vi "PositionControlwithGCompensation.vi"() -> ()   [LabVIEW 2019]
uses:
  <vilib>/myRIO/Common/Instrument Driver Framework/myRIO v1.0/Encoder/typedefs/Encoder Signal Mode.ctl
  <vilib>/myRIO/Instrument Drivers/Onboard IO/Encoder/typedefs/Encoder Reference.ctl
  <vilib>/myRIO/Common/Instrument Driver Framework/Utilities/typedefs/myRIO Generic Hardware Reference.ctl
  <vilib>/myRIO/Common/Instrument Driver Framework/Utilities/typedefs/Hardware Version Enum.ctl
  <vilib>/myRIO/Common/Instrument Driver Framework/Utilities/typedefs/myRIO v1.0 Reference.ctl
  <vilib>/myRIO/Common/Instrument Driver Framework/Utilities/typedefs/Generic FPGA Reference.ctl
  <vilib>/myRIO/Common/Instrument Driver Framework/myRIO v1.0/Encoder/typedefs/Encoder Channels Enum.ctl
  <vilib>/myRIO/Common/Instrument Driver Framework/myRIO v1.0/Encoder/typedefs/Encoder Configuration v1.0.ctl
  <vilib>/userDefined/High Color/nirio_resource_hc.ctl
  <vilib>/myRIO/Common/Instrument Driver Framework/Utilities/vis/Is FPGA Ref Available.vi
  <vilib>/myRIO/Common/Instrument Driver Framework/myRIO v1.0/Encoder/vis/myRIO v1.1 Open Encoder.vi
  <vilib>/myRIO/Instrument Drivers/Onboard IO/Encoder/vis/Read.vi
  <vilib>/myRIO/Common/Instrument Driver Framework/Utilities/vis/Validate Channels.vi
  <vilib>/myRIO/Common/Instrument Driver Framework/myRIO v1.0/Encoder/vis/myRIO v1.0 Reserve Encoder.vi
  <vilib>/myRIO/Common/Instrument Driver Framework/myRIO v1.0/UART/vis/myRIO v1.0 Close UART.vi
  <vilib>/myRIO/Common/Instrument Driver Framework/myRIO v1.0/Encoder/vis/myRIO v1.0 Build MUX Configuration Encoder.vi
  <vilib>/myRIO/Common/Instrument Driver Framework/myRIO v1.0/Resource Manager/vis/myRIO v1.0 Reserve Channel List.vi
  <vilib>/myRIO/Common/Instrument Driver Framework/myRIO v1.0/Resource Manager/vis/myRIO v1.0 Create Configuration List.vi
  <vilib>/myRIO/Common/Instrument Driver Framework/myRIO v1.0/Resource Manager/vis/myRIO v1.0 Reserve Channel.vi
  <vilib>/myRIO/Common/Instrument Driver Framework/myRIO v1.0/Resource Manager/vis/myRIO v1.0 Unreserve Channel.vi
  <vilib>/myRIO/Common/Instrument Driver Framework/myRIO v1.0/Resource Manager/vis/myRIO v1.0 Build Mutex Name.vi
  <vilib>/Utility/VariantDataType/GetNumericInfo.vi
  <vilib>/Utility/error.llb/Error Cluster From Error Code.vi
  <vilib>/myRIO/Common/Instrument Driver Framework/myRIO v1.0/myRIO v1.1 Open.vi
  <vilib>/myRIO/Common/Instrument Driver Framework/Utilities/vis/IO Manager.vi
  <vilib>/myRIO/Common/Instrument Driver Framework/Utilities/vis/Configuration Manager.vi
  <vilib>/myRIO/Common/Instrument Driver Framework/myRIO v1.0/Resource Manager/vis/myRIO v1.0 Configure IO.vi
  <vilib>/myRIO/Common/Instrument Driver Framework/myRIO v1.0/myRIO v1.0 Close.vi
  <vilib>/myRIO/Common/Instrument Driver Framework/myRIO v1.0/Encoder/vis/myRIO v1.0 Configure Encoder.vi
  <vilib>/myRIO/Common/Instrument Driver Framework/myRIO v1.0/Encoder/vis/myRIO v1.0 Read Encoder.vi
  <vilib>/Utility/file.llb/Write Delimited Spreadsheet (DBL).vi
  <vilib>/myRIO/Common/Instrument Driver Framework/Utilities/vis/FPGA Ref Manager.vi
  <vilib>/myRIO/Common/Instrument Driver Framework/myRIO v1.0/myRIO v1.0 Reset FPGA.vi
  <vilib>/myRIO/Common/Instrument Driver Framework/myRIO v1.0/IRQ/vis/myRIO v1.0 IRQ Info FGV.vi
  <vilib>/myRIO/Common/Instrument Driver Framework/myRIO v1.0/IRQ/vis/myRIO v1.0 Timer IRQ Info FGV.vi
  <vilib>/myRIO/Common/Instrument Driver Framework/myRIO v1.0/IRQ/vis/myRIO v1.0 ISR Agent.vi
  <vilib>/myRIO/Instrument Drivers/Utilities/vis/Reset Index.vi
  <vilib>/myRIO/Common/Instrument Driver Framework/myRIO v1.0/Resource Manager/vis/myRIO v1.0 Block Write Resource Manager.vi
  <vilib>/myRIO/Express VI/Onboard IO/Encoder/Encoder Express VI.xnode
  <vilib>/myRIO/Common/Instrument Driver Framework/myRIO v1.0/Encoder/typedefs/Encoder Count Direction Enum.ctl
  <vilib>/myRIO/Instrument Drivers/Onboard IO/Encoder/vis/myRIO Encoder Open.xnode
  <vilib>/myRIO/Instrument Drivers/Onboard IO/Encoder/Encoder.lvlib
  <vilib>/myRIO/Instrument Drivers/Utilities/Utilities.lvlib
panel:
  out "error out 2":errorcluster
  in  "Stop 2":bool
  out "Counter Direction":enum16{"Counting Up", "Counting Down"}(ring)
  out "Overflow?":bool
  in  "Reset Counter":bool
  out "actual pos":dbl
  out "Graph":cluster{dbl, dbl}(graph)
  in  "Frequency [Hz]":dbl=1000.0
  out "Duty Cycle":dbl=0.5
  in  "k_":dbl
  in  "b_":dbl=1.0
  in  "reference":dbl
  out "K1_c":dbl
  out "K2_c":dbl
  out "target pos":dbl
  out "Graph 2":dbl(graph)
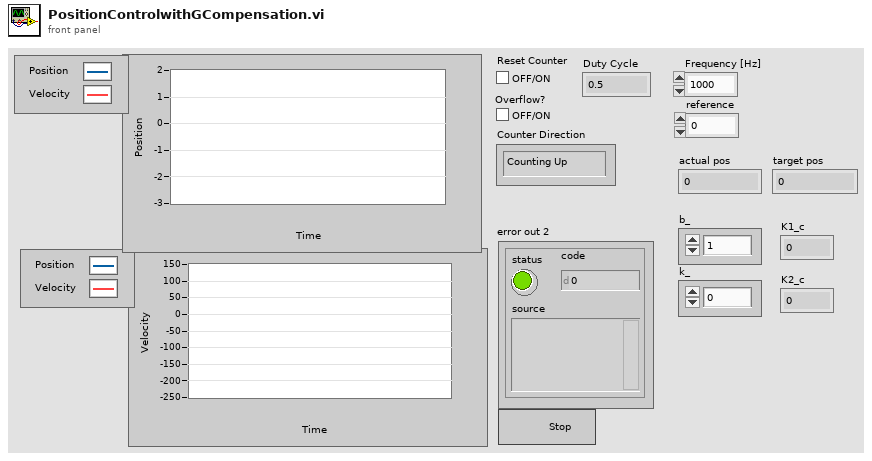
[diagram p1: front panel]
types:
  T1 = typedef "Encoder.lvlib/Encoder Reference.ctl" = cluster{"myRIO Reference":T2, "Encoder Channels Enum":T6}
  T2 = typedef "myRIO Generic Hardware Reference.ctl" = cluster{"myRIO Model":T3, "myRIO Hardware Reference":T4}
  T3 = typedef "Hardware Version Enum.ctl" = enum16{"Unknown", "myRIO-1900", "myRIO-1950", "roboRIO", "NI ELVIS RIO CM", "ELVIS III"}
  T4 = typedef "myRIO v1.0 Reference.ctl" = cluster{"Generic FPGA Reference":T5, "Allow multiple opens":bool}
  T5 = typedef "Generic FPGA Reference.ctl" = refnum<k20>
  T6 = typedef "Encoder Channels Enum.ctl" = enum16{"Not Connected", "C/ENC0", "C/ENC1", "A/ENC", "A/ENC0", "A/ENC1", "A/ENC2", "A/ENC3", "A/ENC4", "A/ENC5", "A/ENC6", "A/ENC7", "A/ENC8", "A/ENC9", "B/ENC", "B/ENC0", "B/ENC1", "B/ENC2", "B/ENC3", "B/ENC4", "B/ENC5", "B/ENC6", "B/ENC7", "B/ENC8", "B/ENC9", "DIO/ENC0", "DIO/ENC1", "DIO/ENC2", "DIO/ENC3", "DIO/ENC4"}
  T7 = typedef "Encoder Signal Mode.ctl" = enum16{"Quadrature phase signal", "Step and direction signal"}
  T8 = typedef "nirio_resource_hc.ctl" = tag
  T9 = typedef "Encoder Count Direction Enum.ctl" = enum16{"Counting Up", "Counting Down"}
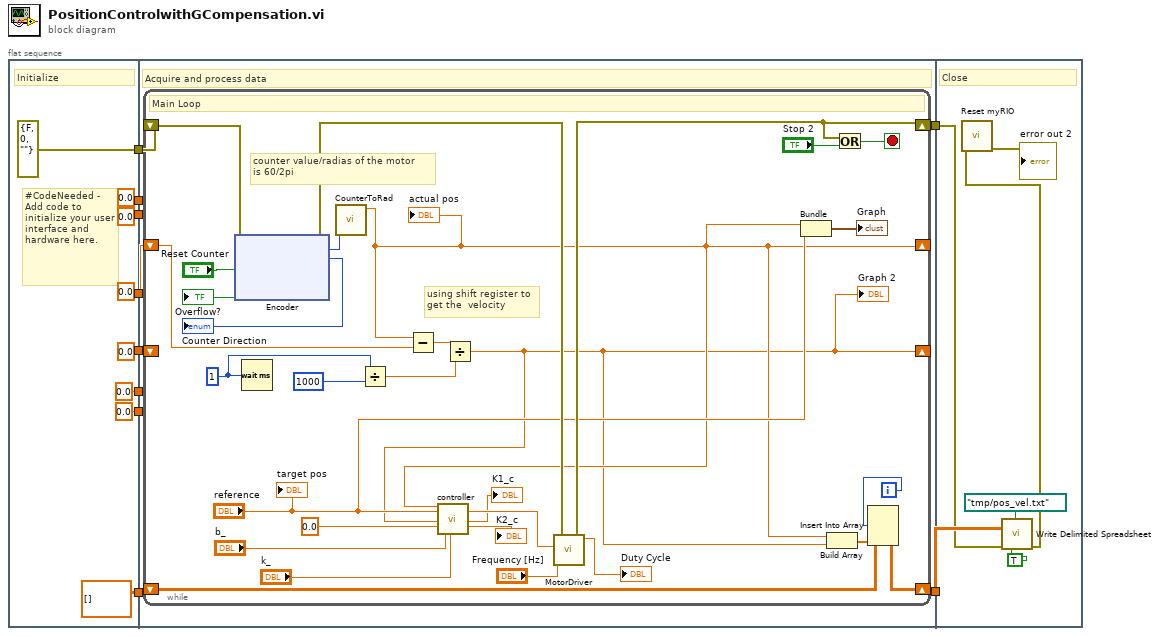
[diagram p0: block diagram]
diagram:
  n1 = flat-sequence {
    tunnel: [errorcluster {"status"=FALSE, "code"=0, "source"=""} ("error in (no error)")] -> w10
    tunnel: [0.0] -> w9
    tunnel: [dbl[][] [] ("array")] -> w8
    tunnel: [0.0] -> w7
    tunnel: [0.0] -> w6
    tunnel: [0.0] -> w5
    tunnel: [0.0 ("Buffer out")] -> w4
    tunnel: [0.0 ("Sum out")] -> w3
    tunnel: w10 -> [w24]
    tunnel: w9 -> [w23]
    tunnel: w8 -> [w22]
    tunnel: w7 -> [w21]
    tunnel: [w20] -> w2
    tunnel: [w19] -> w1
    tunnel: w6 -> [_]
    tunnel: w5 -> [_]
    tunnel: w4 -> [_]
    tunnel: w3 -> [_]
    tunnel: w2 -> [w105]
    tunnel: w1 -> [w104]
    frame #0 {
      # "#CodeNeeded - Add code to initialize your user interface and hardware here."
      # "Initialize"
    }
    frame #1 {
      # "Acquire and process data"
      n2 = while {
        shift-right: [w39] -> w19
        shift-left: w24 -> [w37]
        shift-right: [w26] -> _
        shift-left: w23 -> [w36]
        shift-right: [w45] -> w20
        shift-left: w22 -> [w44]
        shift-right: [w25] -> _
        shift-left: w21 -> [_]
        i -> [w28]
        stop <- w53 stop-if-true
        w49 = u32 1 ("milliseconds to wait")
        # "using shift register to\nget the  velocity"
        # "counter value/radias of the motor \nis 60/2pi"
        # "Main Loop"
        n3 = xnode "Encoder"("error in (no error)"=w37, "Reset Counter"="Reset Counter") -> ("error out"=w40:errorcluster, "Counter Value"=w46:i32, "Counter Direction"=→"Counter Direction":T9, "Overflow?"=→"Overflow?":bool)
        n4 = Wait (ms)(milliseconds to wait=w49) -> ()  [unwired: 1 out]
        n5 = call "CounterToRad.vi"("Counter Value"=w46) -> ("rads"=w26:dbl)  [unwired: 10 in]
        "actual pos" <- w26
        n6 = Divide(x=w49, y=u32 1000) -> (x/y=w38:dbl)
        n7 = Subtract(x=w26, y=w36) -> (x-y=w47:dbl)
        n8 = Divide(x=w47, y=w38) -> (x/y=w25:dbl)
        "Graph 2" <- w25
        n9 = call "controller.vi"("position"=w26, "pos ref"="reference", "velocity"=w25, "vel ref"=0.0, "b_"="b_", "k_"="k_") -> ("duty out"=w35:dbl, "K1_c"=→"K1_c":dbl, "K2_c"=→"K2_c":dbl)  [unwired: 11 in]
        n10 = call "MotorDriver.vi"("error in (no error)"=w40, "Duty Cycle in"=w35, "Frequency [Hz]"="Frequency [Hz]") -> ("error out"=w39:errorcluster, "Duty Cycle out"=→"Duty Cycle":dbl)  [unwired: 7 in]
        n11 = Bundle("rads"=w26, "reference"="reference") -> (→"Graph":cluster{"rads":dbl, "reference":dbl})  [unwired: 1 in]
        n12 = Build Array(w26, w25) -> (w43:dbl[])
        n13 = Or(x=w39, y="Stop 2") -> (x .or. y?=w53:bool)
        n14 = Insert Into Array(array=w44, index (row)=w28, new element=w43) -> (w45:dbl[][])  [unwired: 1 in]
        "target pos" <- "reference"
      }
    }
    frame #2 {
      # "Close"
      n15 = call-poly <vilib>:"Write Delimited Spreadsheet.vi"("file path (dialog if empty)"=path "/tmp/pos_vel.txt", "2D data"=w105, "error in (no error)"=w104, "transpose? (no:F)"=TRUE) -> ("error out"=w103:errorcluster)  [unwired: 10 in, 1 out]
      n16 = call <vilib>:"Reset myRIO.vi"("error in (no error)"=w103) -> ("error out"=→"error out 2":errorcluster)  [unwired: 10 in]
    }
  }
